vi "subVI QCam Set Exposures.vi"(0 "qExposure":dbl=0.4, 1 "qExposure Red":dbl=0.4, 2 "cameraId In":u32, 3 "error In":errorcluster, 4 "qExposure Blue":dbl=0.4, 6 "Set Which Exposure":enum16{"All", "Green", "Red", "Blue"}(ring)=enum."Green") -> (5 "cameraId out":u32, 7 "error out":errorcluster)   [LabVIEW 2012]
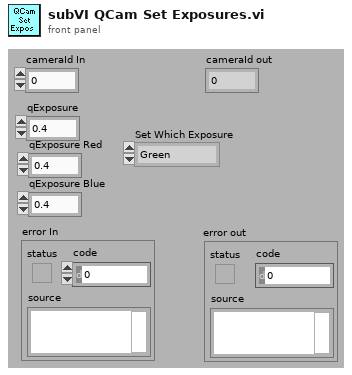
[diagram p1: front panel]
types:
  T1 = enum32{"gain", "offset", "exposure", "binning", "horizontal binning", "vertical binning", "readout speed", "trigger type", "lcd filter", "cooler", "exposure red", "exposure blue", "image format", "roi x", "roi y", "roi width", "roi height", "reserved1", "shutter state", "reserved2", "sync-b out", "reserved3", "intensifier gain", "trigger delay", "camera mode", "normalized gain", "normalized intenifier gain DB", "doPostProcessing", "postProcessGainRed", "postProcessGainGreen", "postProcessGainBlue", "postProcessBayerAlgorithm", "postProcessImageFormat", "fan", "blackout mode", "high sensitivity", "Readout Port", "EM Gain", "open delay", "close delay", "clearing mode"}
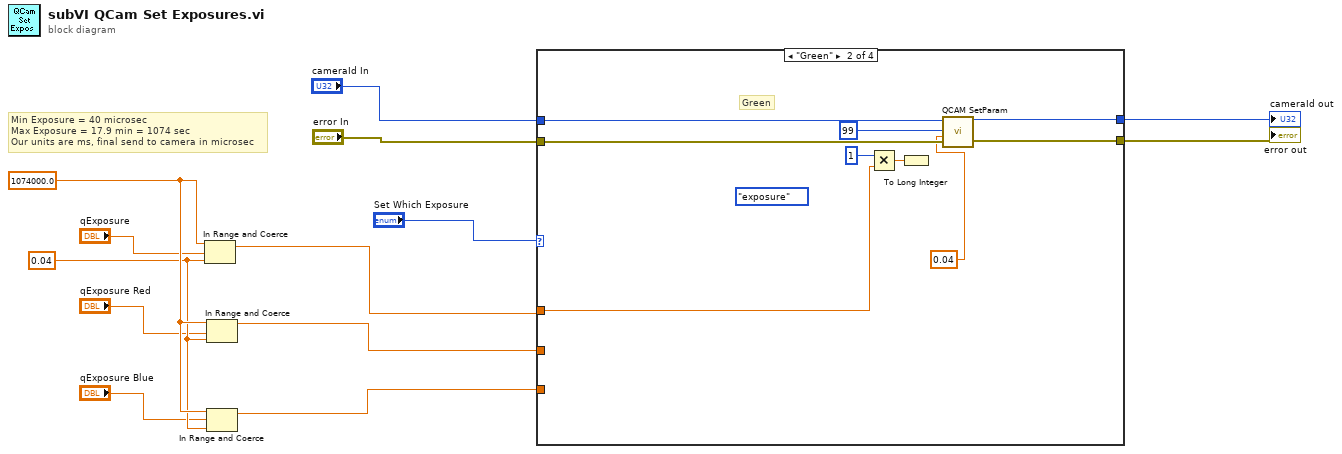
[diagram p0: block diagram]
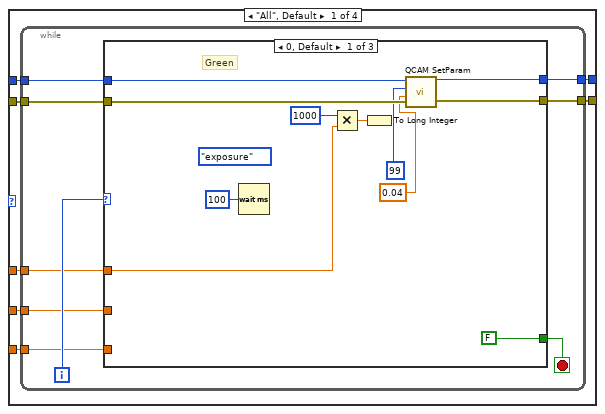
[diagram p2: hidden frame]
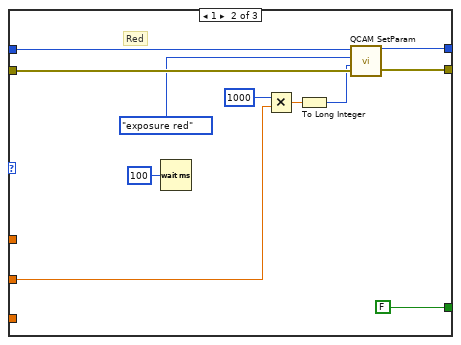
[diagram p3: hidden frame]
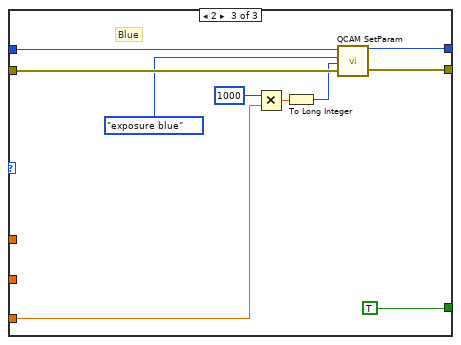
[diagram p4: hidden frame]
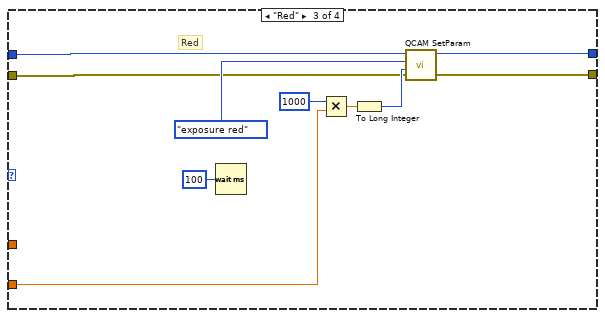
[diagram p5: hidden frame]
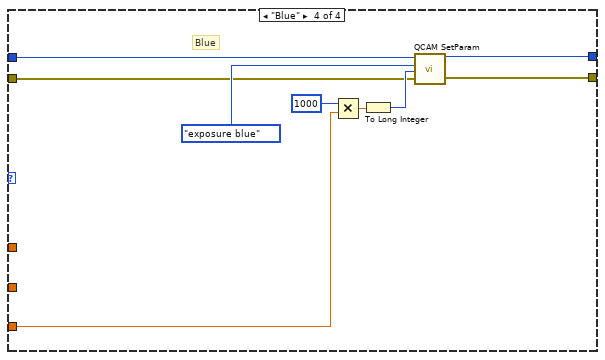
[diagram p6: hidden frame]
diagram:
  w7 = 0.04 ("lower limit")
  w8 = 1074000.0 ("upper limit")
  # "Min Exposure = 40 microsec\nMax Exposure = 17.9 min = 1074 sec\nOur units are ms, final send to camera in microsec"
  n1 = In Range and Coerce(upper limit=w8, x="qExposure", lower limit=w7) -> (coerced(x)=w3:dbl)  [unwired: 1 out]
  n2 = In Range and Coerce(upper limit=w8, x="qExposure Red", lower limit=w7) -> (coerced(x)=w2:dbl)  [unwired: 1 out]
  n3 = In Range and Coerce(upper limit=w8, x="qExposure Blue", lower limit=w7) -> (coerced(x)=w1:dbl)  [unwired: 1 out]
  n4 = case shown="\"Green\"" "Set Which Exposure" {
    tunnel: [w20 w66 w72 w83] -> w13
    tunnel: [w19 w65 w73 w82] -> w12
    tunnel: "error In" -> [w18 w68 w74 w84]
    tunnel: "cameraId In" -> [w17 w67 w75 w85]
    tunnel: w3 -> [w16 w64 _ _]
    tunnel: w2 -> [w15 _ w71 _]
    tunnel: w1 -> [w14 _ _ w81]
    frame "All", Default {
      n5 = while {
        tunnel: w17 -> [w28]
        tunnel: w18 -> [w27]
        tunnel: [w25] -> w19
        tunnel: [w24] -> w20
        tunnel: w16 -> [w23]
        tunnel: w15 -> [w22]
        tunnel: w14 -> [w21]
        i -> [w29]
        stop <- w26 stop-if-true
        n6 = case shown="0, Default" w29 {
          tunnel: w28 -> [w39 w50 w60]
          tunnel: w27 -> [w37 w48 w58]
          tunnel: [FALSE FALSE TRUE] -> w26
          tunnel: [w36 w47 w57] -> w25
          tunnel: [w38 w49 w59] -> w24
          tunnel: w23 -> [w32 _ _]
          tunnel: w22 -> [_ w41 _]
          tunnel: w21 -> [_ _ w52]
          frame 0, Default {
            (unwired) T1."exposure" ("parameter key")
            # "Green"
            n7 = Wait (ms)(milliseconds to wait=u32 100) -> ()  [unwired: 1 out]
            n8 = Multiply(x=u32 1000, y=w32) -> (x*y=w33:dbl)
            n9 = To Long Integer(number=w33) -> ()  [unwired: 1 out]
            n10 = call "QCAM SetParam.vi"("error in (no error)"=w37, "value"=0.04 ("lower limit"), "parameter key"=u32 99 ("milliseconds to wait"), "cameraId"=w39) -> ("error out"=w36:errorcluster, "cameraId out"=w38:u32)
          }
          frame 1 {
            # "Red"
            n11 = Wait (ms)(milliseconds to wait=u32 100) -> ()  [unwired: 1 out]
            n12 = Multiply(x=u32 1000, y=w41) -> (x*y=w43:dbl)
            n13 = To Long Integer(number=w43) -> (32bit integer=w42:i32)
            n14 = call "QCAM SetParam.vi"("error in (no error)"=w48, "value"=w42, "parameter key"=T1."exposure red", "cameraId"=w50) -> ("error out"=w47:errorcluster, "cameraId out"=w49:u32)
          }
          frame 2 {
            # "Blue"
            n15 = Multiply(x=u32 1000, y=w52) -> (x*y=w54:dbl)
            n16 = To Long Integer(number=w54) -> (32bit integer=w53:i32)
            n17 = call "QCAM SetParam.vi"("error in (no error)"=w58, "value"=w53, "parameter key"=T1."exposure blue", "cameraId"=w60) -> ("error out"=w57:errorcluster, "cameraId out"=w59:u32)
          }
        }
      }
    }
    frame "Green" {
      (unwired) T1."exposure" ("parameter key")
      # "Green"
      n18 = Multiply(x=u32 1, y=w64) -> (x*y=w69:dbl)
      n19 = To Long Integer(number=w69) -> ()  [unwired: 1 out]
      n20 = call "QCAM SetParam.vi"("error in (no error)"=w68, "value"=0.04 ("lower limit"), "parameter key"=u32 99 ("x"), "cameraId"=w67) -> ("error out"=w65:errorcluster, "cameraId out"=w66:u32)
    }
    frame "Red" {
      # "Red"
      n21 = Wait (ms)(milliseconds to wait=u32 100) -> ()  [unwired: 1 out]
      n22 = Multiply(x=u32 1000, y=w71) -> (x*y=w77:dbl)
      n23 = To Long Integer(number=w77) -> (32bit integer=w76:i32)
      n24 = call "QCAM SetParam.vi"("error in (no error)"=w74, "value"=w76, "parameter key"=T1."exposure red", "cameraId"=w75) -> ("error out"=w73:errorcluster, "cameraId out"=w72:u32)
    }
    frame "Blue" {
      # "Blue"
      n25 = Multiply(x=u32 1000, y=w81) -> (x*y=w87:dbl)
      n26 = To Long Integer(number=w87) -> (32bit integer=w86:i32)
      n27 = call "QCAM SetParam.vi"("error in (no error)"=w84, "value"=w86, "parameter key"=T1."exposure blue", "cameraId"=w85) -> ("error out"=w82:errorcluster, "cameraId out"=w83:u32)
    }
  }
  "cameraId out" <- w13
  "error out" <- w12
